vi "Get Specific Filter Configuration String.vi"(11 "Boolean Filter in":refnum<class "Boolean Filter.lvclass">) -> (2 "Filter String":string)   [LabVIEW 2017, in "Assert API Components.lvlib" / "Boolean Filter.lvclass"]
uses:
  Boolean Filter.lvclass
  Boolean Filter.lvclass/Boolean Filter.ctl
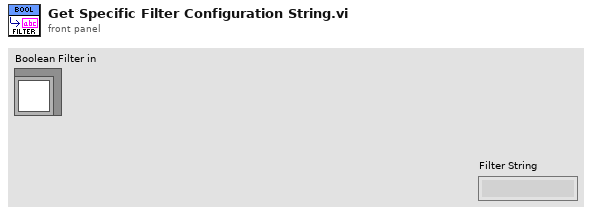
[diagram p1: front panel]
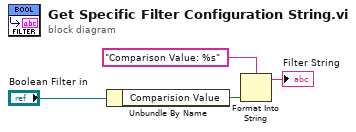
[diagram p0: block diagram]
diagram:
  n1 = Unbundle By Name("Boolean Filter in") -> ("Comparision Value"=w3:bool)
  n2 = Format Into String(format string="Comparison Value: %s", w3) -> (resulting string=→"Filter String":string)  [unwired: 2 in, 1 out]
